vi "Teleop.vi"(10 "Match Info":T1={"Autonomous Elapsed Seconds"=0.0, "TeleOp Elapsed Seconds"=0.0, "Disabled Elapsed Seconds"=0.0, "Visited Autonomous"=FALSE, "Visited TeleOp"=FALSE, "Visited Disabled"=FALSE, "Autonomous Settings"={"Autonomous Style"=enum."Independent", "VI Refnum"=refnum}}, 11 "Call Context":T2) -> ()   [LabVIEW 2011]
doc: "This VI is called for each TeleOp packet received from the DS where the robot is not disabled. It is often used to read from the joysticks and update I/O or to update setpoints for timed control loops. It should complete and return within 20 milliseconds or it may miss DS packets."
uses:
  <vilib>/Rock Robotics/WPI/DriverStation/WPI_DriverStationDerivedRobotMode.ctl
  <vilib>/Rock Robotics/WPI/DriverStation/WPI_DriverStationMatch Info.ctl
  <vilib>/Rock Robotics/WPI/Relay/WPI_RelayValue.ctl
  <vilib>/Rock Robotics/WPI/DriverStation/DriverStationLCD/WPI_DriverStationLCDLCDLine.ctl
  Robot Global Data.vi
panel:
  in  "LDrive0":dbl
  in  "Rdrive0":dbl=0.9
  in  "Rdrive2":dbl=0.6
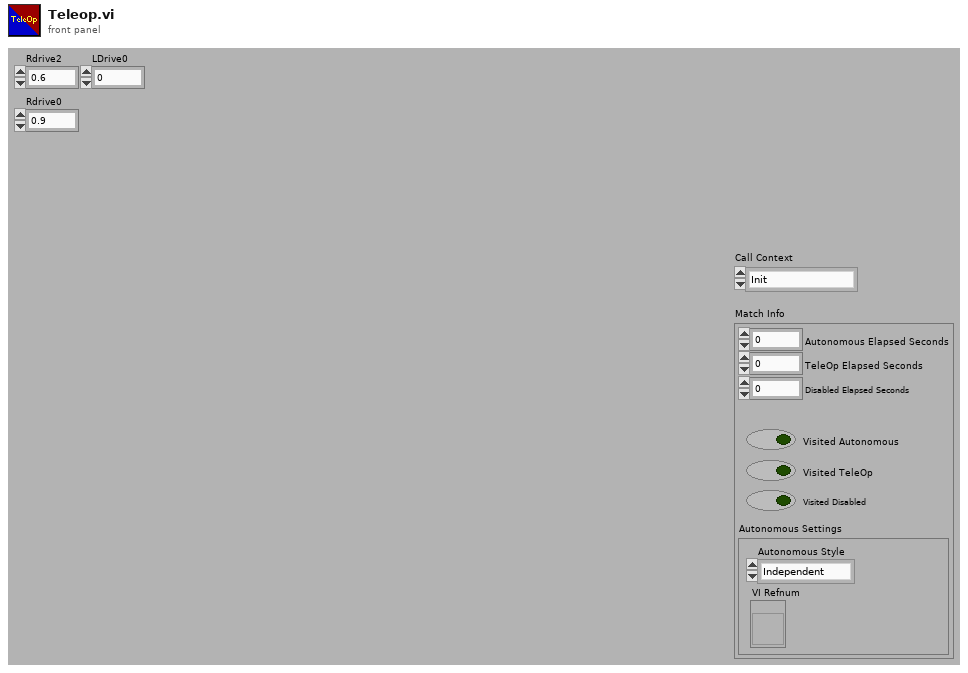
[diagram p1: front panel]
types:
  T1 = typedef "WPI_DriverStationMatch Info.ctl" = cluster{"Autonomous Elapsed Seconds":dbl, "TeleOp Elapsed Seconds":dbl, "Disabled Elapsed Seconds":dbl, "Visited Autonomous":bool, "Visited TeleOp":bool, "Visited Disabled":bool, "Autonomous Settings":cluster{"Autonomous Style":enum16{"Iterative", "Independent"}, "VI Refnum":refnum<vi>}}
  T2 = typedef "WPI_DriverStationDerivedRobotMode.ctl" = enum16{"Init", "Execute", "Stop"}
  T3 = typedef "WPI_RelayValue.ctl" = enum16{"Off", "On", "Forward", "Reverse"}
  T4 = typedef "WPI_JoystickDevRef.ctl" = cluster{"Device":T5}
  T5 = typedef "WPI_JoystickDeviceEnum.ctl" = enum16{"USB 1", "USB 2", "USB 3", "USB 4", "Kinect 1", "Kinect 2"}
  T6 = typedef "WPI_JoystickButtonState.ctl" = cluster{"Button 1":bool, "Button 2":bool, "Button 3":bool, "Button 4":bool, "Button 5":bool, "Button 6":bool, "Button 7":bool, "Button 8":bool, "Button 9":bool, "Button 10":bool, "Button 11":bool, "Button 12":bool}
  T7 = cluster{"axis 1 (x)":dbl, "axis 2 (y)":dbl, "axis 3 (throttle)":dbl, "axis 4":dbl, "axis 5":dbl, "axis 6":dbl}
  T8 = typedef "WPI_MotorControlDeviceRef.ctl" = cluster{"DeviceStatus":errorcluster, "Type":enum16{"PWM", "CAN"}, "PWM":cluster{"Digital Module":T9, "PWM Channel":T10, "DeadBand":T11}, "CAN":cluster{"Device Number":u8, "Control Mode":T12, "Semaphore":T13, "Max Vout":dbl}, "Invert":bool, "TransformRef":T14, "InvTransformRef":T14}
  T9 = typedef "FPGA_TypedefDigitalModule.ctl" = enum16{"Digital Module 1", "Digital Module 2"}
  T10 = typedef "FPGA_DIOPWMChannel.ctl" = enum8{"PWM 1", "PWM 2", "PWM 3", "PWM 4", "PWM 5", "PWM 6", "PWM 7", "PWM 8", "PWM 9", "PWM 10", "Invalid"}
  T11 = typedef "WPI_PWMDeadband.ctl" = cluster{"Name":string, "maxPositivePwm":i32, "minPositivePwm":i32, "centerPwm":i32, "maxNegativePwm":i32, "minNegativePwm":i32, "angularRange":u16}
  T12 = typedef "WPI_CANJaguar_ControlMode.ctl" = enum8{"Percent VBus", "Current", "Speed", "Position", "Voltage"}
  T13 = typedef "Semaphore RefNum" = refnum<k1>
  T14 = typedef "WPI_PWMTransform_ConPane.ctl" = refnum<vi>
  T15 = cluster{"Driver Station Digital Input (1-8)[0]":bool, "Driver Station Digital Input (1-8)[1]":bool, "Driver Station Digital Input (1-8)[2]":bool, "Driver Station Digital Input (1-8)[3]":bool, "Driver Station Digital Input (1-8)[4]":bool, "Driver Station Digital Input (1-8)[5]":bool, "Driver Station Digital Input (1-8)[6]":bool, "Driver Station Digital Input (1-8)[7]":bool, "Driver Station Digital Input (1-8)[8]":bool}
  T16 = typedef "WPI_RelayDevRef.ctl" = cluster{"DevStatus":errorcluster, "Relay Channel":T17, "Digital Module":T9, "Relay Direction":T18}
  T17 = typedef "FPGA_DIORelayChannel.ctl" = enum8{"Relay 1", "Relay 2", "Relay 3", "Relay 4", "Relay 5", "Relay 6", "Relay 7", "Relay 8", "Invalid"}
  T18 = typedef "WPI_RelayDirection.ctl" = enum16{"Both directions", "Forward only", "Reverse only"}
  T19 = typedef "WPI_DigitalInputDevRef.ctl" = cluster{"DevStatus":errorcluster, "DIO Channel":T20, "Digital Module":T9}
  T20 = typedef "FPGA_DIOChannel.ctl" = enum8{"DIO 1", "DIO 2", "DIO 3", "DIO 4", "DIO 5", "DIO 6", "DIO 7", "DIO 8", "DIO 9", "DIO 10", "DIO 11", "DIO 12", "DIO 13", "DIO 14", "Invalid"}
  T21 = typedef "WPI_EncoderDevRef.ctl" = cluster{"DevStatus":errorcluster, "EncoderIndex":T22, "CounterIndex":T23, "DistancePerCount":dbl, "Decoding Type":T24}
  T22 = typedef "FPGA_EncoderIdx.ctl" = enum8{"Enc 0", "Enc 1", "Enc 2", "Enc 3", "Invalid"}
  T23 = typedef "FPGA_CounterCtrSystemIndex.ctl" = enum8{"Ctr 0", "Ctr 1", "Ctr 2", "Ctr 3", "Ctr 4", "Ctr 5", "Ctr 6", "Ctr 7", "Invalid"}
  T24 = typedef "WPI_EncoderType.ctl" = enum16{"1x", "2x", "4x"}
  T25 = typedef "WPI_DriverStationLCDLCDLine.ctl" = enum16{"Main - Line 1", "User - Line 2", "User - Line 3", "User - Line 4", "User - Line 5", "User - Line 6"}
  T26 = typedef "WPI_ServoDeviceRef.ctl" = cluster{"DeviceStatus":errorcluster, "Digital Module":T9, "PWM Channel":T10, "DeadBand":T11}
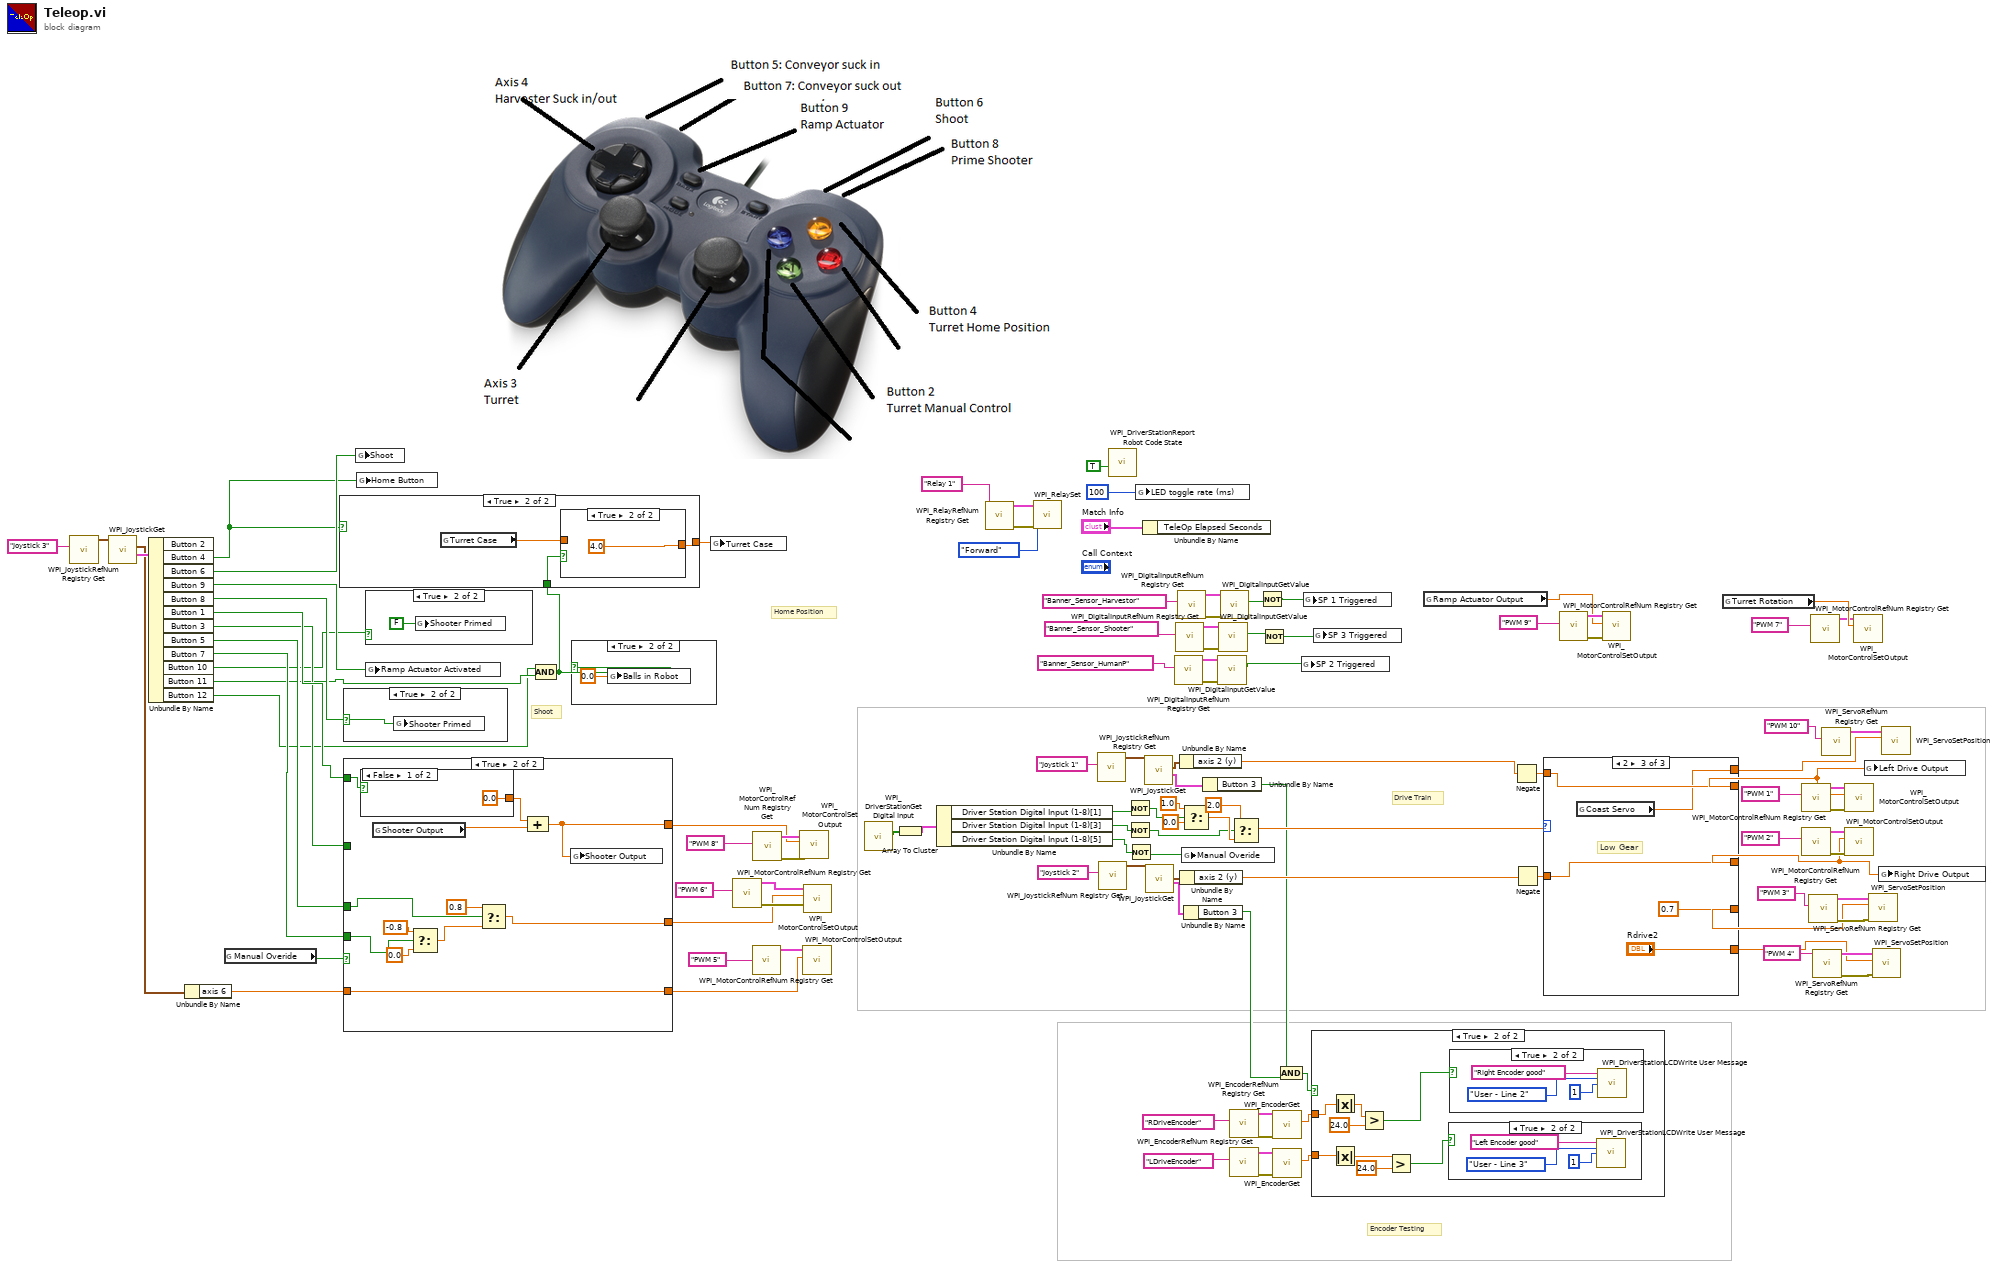
[diagram p0: block diagram]
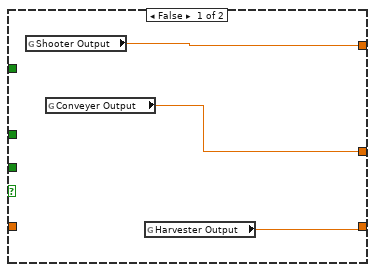
[diagram p7: hidden frame]
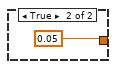
[diagram p8: hidden frame]
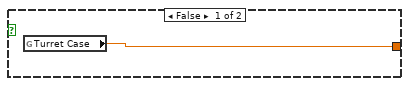
[diagram p10: hidden frame]
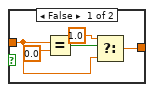
[diagram p11: hidden frame]
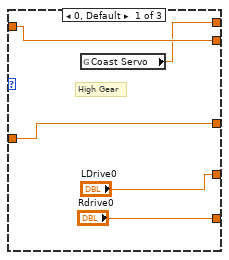
[diagram p12: hidden frame]
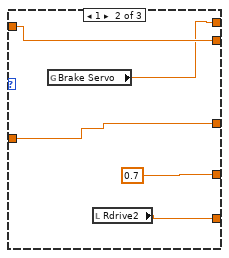
[diagram p13: hidden frame]
diagram:
  # "Encoder Testing"
  # "Shoot"
  # "Home Position"
  # "Drive Train"
  n1 = call <vilib>:"WPI_JoystickRefNum Registry Get.vi"("refnum name"="Joystick 3") -> ("JoystickDevRef"=w66:T4)  [unwired: 9 in, 1 out]
  n2 = call <vilib>:"WPI_JoystickGet.vi"("JoystickDevRef"=w66) -> ("Buttons"=w67:T6, "Axes"=w40:T7)  [unwired: 4 in, 1 out]
  n3 = Unbundle By Name(w67) -> ("Button 4"=w25:bool, "Button 6"=w65:bool, "Button 9"=w69:bool, "Button 8"=w41:bool, "Button 1"=w27:bool, "Button 3"=w26:bool, "Button 5"=w35:bool, "Button 7"=w34:bool, "Button 10"=w24:bool, "Button 11"=w23:bool, "Button 12"=w22:bool)  [unwired: 1 out]
  n4 = Unbundle By Name(w40) -> ("axis 6"=w20:dbl)
  n5 = global read "Robot Global Data.vi" "Manual Overide"() -> (w29:bool)
  n6 = case shown="True" w41 {
    selector: w41 -> [_ w114]
    frame False {
    }
    frame True {
      n7 = global write "Robot Global Data.vi" "Shooter Primed"(w114) -> ()
    }
  }
  n8 = case shown="True" w29 {
    tunnel: [w117 w119] -> w36
    tunnel: w27 -> [_ w122]
    tunnel: w26 -> [_ _]
    tunnel: w35 -> [_ w124]
    tunnel: w34 -> [_ w125]
    tunnel: [w116 w123] -> w30
    tunnel: [w115 w118] -> w21
    tunnel: w20 -> [_ w118]
    frame False {
      n9 = global read "Robot Global Data.vi" "Shooter Output"() -> (w117:dbl)
      n10 = global read "Robot Global Data.vi" "Conveyer Output"() -> (w116:dbl)
      n11 = global read "Robot Global Data.vi" "Harvester Output"() -> (w115:dbl)
    }
    frame True {
      n12 = case shown="False" w122 {
        tunnel: [0.0 0.05] -> w121
        frame False {
        }
        frame True {
        }
      }
      n13 = global read "Robot Global Data.vi" "Shooter Output"() -> (w120:dbl)
      n14 = Select(t=-0.8, s=w125, f=0.0) -> (s? t:f=w129:dbl)
      n15 = Select(t=0.8, s=w124, f=w129) -> (s? t:f=w123:dbl)
      n16 = Compound Arithmetic op=ADD(w121, w120) -> (w119:dbl)
      n17 = global write "Robot Global Data.vi" "Shooter Output"(w119) -> ()
    }
  }
  n18 = global write "Robot Global Data.vi" "Shoot"(w65) -> ()
  n19 = global write "Robot Global Data.vi" "Home Button"(w25) -> ()
  n20 = case shown="True" w24 {
    frame False {
    }
    frame True {
      n21 = global write "Robot Global Data.vi" "Shooter Primed"(FALSE ("Shooter Primed")) -> ()
    }
  }
  n22 = global write "Robot Global Data.vi" "Ramp Actuator Activated"(w69) -> ()
  n23 = Compound Arithmetic op=AND(w22, w23) -> (w19:bool)
  n24 = case shown="True" w25 {
    tunnel: [w133 w134] -> w18
    tunnel: w19 -> [_ w136]
    frame False {
      n25 = global read "Robot Global Data.vi" "Turret Case"() -> (w133:dbl)
    }
    frame True {
      n26 = global read "Robot Global Data.vi" "Turret Case"() -> (w135:dbl)
      n27 = case shown="True" w136 {
        tunnel: w135 -> [w138 _]
        tunnel: [w137 4.0 ("Turret Case")] -> w134
        frame False {
          n28 = Equal?(x=w138, y=0.0) -> (x = y?=w140:bool)
          n29 = Select(t=1.0, s=w140, f=w138) -> (s? t:f=w137:dbl)
        }
        frame True {
        }
      }
    }
  }
  n30 = case shown="True" w19 {
    frame False {
    }
    frame True {
      n31 = global write "Robot Global Data.vi" "Balls in Robot"(0.0 ("Balls in Robot")) -> ()
    }
  }
  n32 = global write "Robot Global Data.vi" "Turret Case"(w18) -> ()
  n33 = call <vilib>:"WPI_MotorControlRefNum Registry Get.vi"("refnum name"="PWM 6") -> ("error out"=w31:errorcluster, "MotorControlDevRef"=w32:T8)  [unwired: 9 in]
  n34 = call <vilib>:"WPI_MotorControlRefNum Registry Get.vi"("refnum name"="PWM 5") -> ("MotorControlDevRef"=w59:T8)  [unwired: 9 in, 1 out]
  n35 = call <vilib>:"WPI_MotorControlRefNum Registry Get.vi"("refnum name"="PWM 8") -> ("error out"=w43:errorcluster, "MotorControlDevRef"=w44:T8)  [unwired: 9 in]
  n36 = call <vilib>:"WPI_MotorControlSetOutput.vi"("error in (no error)"=w43, "Output"=w36, "MotorControlDevRef"=w44) -> ()  [unwired: 7 in, 2 out]
  n37 = call <vilib>:"WPI_MotorControlSetOutput.vi"("Output"=w21, "MotorControlDevRef"=w59) -> ()  [unwired: 8 in, 2 out]
  n38 = call <vilib>:"WPI_MotorControlSetOutput.vi"("error in (no error)"=w31, "Output"=w30, "MotorControlDevRef"=w32) -> ()  [unwired: 7 in, 2 out]
  n39 = call <vilib>:"WPI_DriverStationGet Digital Input.vi"() -> ("Driver Station Digital Input (1-8)"=w88:bool[])  [unwired: 11 in]
  n40 = Array To Cluster(array=w88) -> (cluster=w110:T15)
  n41 = Unbundle By Name(w110) -> ("Driver Station Digital Input (1-8)[1]"=w91:bool, "Driver Station Digital Input (1-8)[3]"=w90:bool, "Driver Station Digital Input (1-8)[5]"=w37:bool)
  n42 = call <vilib>:"WPI_RelayRefNum Registry Get.vi"("refnum name"="Relay 1") -> ("error out"=w63:errorcluster, "RelayDevRef"=w64:T16)  [unwired: 9 in]
  n43 = call <vilib>:"WPI_RelaySet.vi"("error in (no error)"=w63, "RelayValue"=WPI_RelayValue."Forward", "RelayDevRef"=w64) -> ()  [unwired: 7 in, 2 out]
  n44 = call <vilib>:"WPI_JoystickRefNum Registry Get.vi"("refnum name"="Joystick 1") -> ("JoystickDevRef"=w103:T4)  [unwired: 9 in, 1 out]
  n45 = call <vilib>:"WPI_JoystickRefNum Registry Get.vi"("refnum name"="Joystick 2") -> ("JoystickDevRef"=w101:T4)  [unwired: 9 in, 1 out]
  n46 = call <vilib>:"WPI_DriverStationReport Robot Code State.vi"("TeleOp"=TRUE ("Autonomous")) -> ()  [unwired: 10 in, 1 out]
  n47 = Not(x=w91) -> (.not. x?=w89:bool)
  n48 = Not(x=w90) -> (.not. x?=w39:bool)
  n49 = Not(x=w37) -> (.not. x?=w38:bool)
  n50 = global write "Robot Global Data.vi" "LED toggle rate (ms)"(u32 100 ("LED ms toggle rate")) -> ()
  n51 = Unbundle By Name("Match Info") -> ()  [unwired: 1 out]
  n52 = call <vilib>:"WPI_JoystickGet.vi"("JoystickDevRef"=w103) -> ("Buttons"=w15:T6, "Axes"=w16:T7)  [unwired: 4 in, 1 out]
  n53 = call <vilib>:"WPI_JoystickGet.vi"("JoystickDevRef"=w101) -> ("Buttons"=w17:T6, "Axes"=w102:T7)  [unwired: 4 in, 1 out]
  n54 = call <vilib>:"WPI_DigitalInputRefNum Registry Get.vi"("refnum name"="Banner_Sensor_HumanP") -> ("error out"=w54:errorcluster, "DigitalInputDevRef"=w53:T19)  [unwired: 9 in]
  n55 = call <vilib>:"WPI_DigitalInputRefNum Registry Get.vi"("refnum name"="Banner_Sensor_Shooter") -> ("error out"=w55:errorcluster, "DigitalInputDevRef"=w56:T19)  [unwired: 9 in]
  n56 = call <vilib>:"WPI_DigitalInputRefNum Registry Get.vi"("refnum name"="Banner_Sensor_Harvestor") -> ("error out"=w58:errorcluster, "DigitalInputDevRef"=w57:T19)  [unwired: 9 in]
  n57 = Unbundle By Name(w16) -> ("axis 2 (y)"=w87:dbl)
  n58 = Unbundle By Name(w102) -> ("axis 2 (y)"=w85:dbl)
  n59 = Select(t=1.0, s=w89, f=0.0 ("t")) -> (s? t:f=w107:dbl)
  n60 = global write "Robot Global Data.vi" "Manual Overide"(w38) -> ()
  n61 = Unbundle By Name(w17) -> ("Button 3"=w13:bool)
  n62 = Unbundle By Name(w15) -> ("Button 3"=w14:bool)
  n63 = call <vilib>:"WPI_DigitalInputGetValue.vi"("error in (no error)"=w54, "DigitalInputDevRef"=w53) -> ("Value"=w49:bool)  [unwired: 7 in, 2 out]
  n64 = call <vilib>:"WPI_DigitalInputGetValue.vi"("error in (no error)"=w55, "DigitalInputDevRef"=w56) -> ("Value"=w48:bool)  [unwired: 7 in, 2 out]
  n65 = call <vilib>:"WPI_DigitalInputGetValue.vi"("error in (no error)"=w58, "DigitalInputDevRef"=w57) -> ("Value"=w46:bool)  [unwired: 7 in, 2 out]
  n66 = call <vilib>:"WPI_EncoderRefNum Registry Get.vi"("refnum name"="RDriveEncoder") -> ("error out"=w9:errorcluster, "EncoderDevRef"=w10:T21)  [unwired: 9 in]
  n67 = call <vilib>:"WPI_EncoderRefNum Registry Get.vi"("refnum name"="LDriveEncoder") -> ("error out"=w8:errorcluster, "EncoderDevRef"=w7:T21)  [unwired: 9 in]
  n68 = Select(t=2.0, s=w39, f=w107) -> (s? t:f=w105:dbl)
  n69 = Not(x=w46) -> (.not. x?=w45:bool)
  n70 = Not(x=w48) -> (.not. x?=w47:bool)
  n71 = call <vilib>:"WPI_EncoderGet.vi"("error in (no error)"=w9, "EncoderDevRef"=w10) -> ("Distance"=w5:dbl)  [unwired: 4 in, 5 out]
  n72 = call <vilib>:"WPI_EncoderGet.vi"("error in (no error)"=w8, "EncoderDevRef"=w7) -> ("Distance"=w4:dbl)  [unwired: 4 in, 5 out]
  n73 = And(x=w14, y=w13) -> (x .and. y?=w12:bool)
  n74 = global write "Robot Global Data.vi" "SP 2 Triggered"(w49) -> ()
  n75 = global write "Robot Global Data.vi" "SP 1 Triggered"(w45) -> ()
  n76 = case shown="True" w12 {
    tunnel: w5 -> [_ w146]
    tunnel: w4 -> [_ w145]
    frame False {
    }
    frame True {
      n77 = Absolute Value(x=w146) -> (abs(x)=w147:dbl)
      n78 = Absolute Value(x=w145) -> (abs(x)=w144:dbl)
      n79 = Greater?(x=w147, y=24.0) -> (0:w150:bool)
      n80 = Greater?(x=w144, y=24.0) -> (0:w148:bool)
      n81 = case shown="True" w148 {
        frame False {
        }
        frame True {
          n82 = call <vilib>:"WPI_DriverStationLCDWrite User Message.vi"("line text"="Left Encoder good", "line"=WPI_DriverStationLCDLCDLine."User - Line 3", "starting column"=i8 1) -> ()  [unwired: 2 in, 11 out]
        }
      }
      n83 = case shown="True" w150 {
        frame False {
        }
        frame True {
          n84 = call <vilib>:"WPI_DriverStationLCDWrite User Message.vi"("line text"="Right Encoder good", "line"=WPI_DriverStationLCDLCDLine."User - Line 2", "starting column"=i8 1) -> ()  [unwired: 2 in, 11 out]
        }
      }
    }
  }
  n85 = global write "Robot Global Data.vi" "SP 3 Triggered"(w47) -> ()
  n86 = global read "Robot Global Data.vi" "Ramp Actuator Output"() -> (w28:dbl)
  n87 = Negate(x=w87) -> (-x=w86:dbl)
  n88 = Negate(x=w85) -> (-x=w84:dbl)
  n89 = case shown="2" w105 {
    tunnel: w84 -> [w162 w165 w172]
    tunnel: [w162 w165 w172] -> w76
    tunnel: [w161 w164 w171] -> w77
    tunnel: ["LDrive0" 0.7 0.7] -> w93
    tunnel: ["Rdrive0" w166 "Rdrive2"] -> w92
    tunnel: w86 -> [w161 w164 w171]
    tunnel: [w158 w163 w168] -> w1
    frame 0, Default {
      # "High Gear"
      n90 = global read "Robot Global Data.vi" "Coast Servo"() -> (w158:dbl)
    }
    frame 1 {
      n91 = global read "Robot Global Data.vi" "Brake Servo"() -> (w163:dbl)
      n92 = local read "Rdrive2"() -> (w166:dbl)
    }
    frame 2 {
      # "Low Gear"
      n93 = global read "Robot Global Data.vi" "Coast Servo"() -> (w168:dbl)
    }
  }
  n94 = call <vilib>:"WPI_MotorControlRefNum Registry Get.vi"("refnum name"="PWM 9") -> ("error out"=w74:errorcluster, "MotorControlDevRef"=w73:T8)  [unwired: 9 in]
  n95 = call <vilib>:"WPI_MotorControlSetOutput.vi"("error in (no error)"=w74, "Output"=w28, "MotorControlDevRef"=w73) -> ()  [unwired: 7 in, 2 out]
  n96 = global read "Robot Global Data.vi" "Turret Rotation"() -> (w72:dbl)
  n97 = call <vilib>:"WPI_MotorControlRefNum Registry Get.vi"("refnum name"="PWM 1") -> ("error out"=w81:errorcluster, "MotorControlDevRef"=w83:T8)  [unwired: 9 in]
  n98 = call <vilib>:"WPI_MotorControlRefNum Registry Get.vi"("refnum name"="PWM 2") -> ("error out"=w80:errorcluster, "MotorControlDevRef"=w79:T8)  [unwired: 9 in]
  n99 = call <vilib>:"WPI_ServoRefNum Registry Get.vi"("refnum name"="PWM 3") -> ("error out"=w97:errorcluster, "ServoDeviceRef"=w98:T26)  [unwired: 9 in]
  n100 = call <vilib>:"WPI_MotorControlRefNum Registry Get.vi"("refnum name"="PWM 7") -> ("MotorControlDevRef"=w70:T8)  [unwired: 9 in, 1 out]
  n101 = call <vilib>:"WPI_ServoRefNum Registry Get.vi"("refnum name"="PWM 4") -> ("error out"=w96:errorcluster, "ServoDeviceRef"=w95:T26)  [unwired: 9 in]
  n102 = call <vilib>:"WPI_ServoRefNum Registry Get.vi"("refnum name"="PWM 10") -> ("ServoDeviceRef"=w3:T26)  [unwired: 9 in, 1 out]
  n103 = call <vilib>:"WPI_MotorControlSetOutput.vi"("error in (no error)"=w81, "Output"=w77, "MotorControlDevRef"=w83) -> ()  [unwired: 7 in, 2 out]
  n104 = call <vilib>:"WPI_MotorControlSetOutput.vi"("error in (no error)"=w80, "Output"=w76, "MotorControlDevRef"=w79) -> ()  [unwired: 7 in, 2 out]
  n105 = call <vilib>:"WPI_MotorControlSetOutput.vi"("Output"=w72, "MotorControlDevRef"=w70) -> ()  [unwired: 8 in, 2 out]
  n106 = global write "Robot Global Data.vi" "Left Drive Output"(w77) -> ()
  n107 = call <vilib>:"WPI_ServoSetPosition.vi"("error in (no error)"=w97, "Position"=w93, "ServoDeviceRef"=w98) -> ()  [unwired: 7 in, 2 out]
  n108 = call <vilib>:"WPI_ServoSetPosition.vi"("error in (no error)"=w96, "Position"=w92, "ServoDeviceRef"=w95) -> ()  [unwired: 7 in, 2 out]
  n109 = global write "Robot Global Data.vi" "Right Drive Output"(w76) -> ()
  n110 = call <vilib>:"WPI_ServoSetPosition.vi"("Position"=w1, "ServoDeviceRef"=w3) -> ()  [unwired: 8 in, 2 out]
